vi "Calculator-V1.2.vi"() -> ()   [LabVIEW 2014]
panel:
  out "Result":dbl
  in  "Equal":bool
  in  "MUL":bool
  in  "SUB":bool
  in  "DEV":bool
  in  "SUM":bool
  in  "y":dbl
  in  "x":dbl
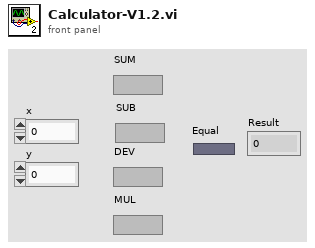
[diagram p1: front panel]
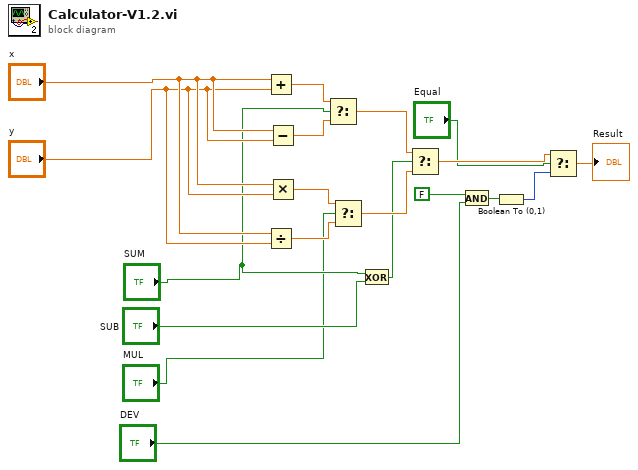
[diagram p0: block diagram]
diagram:
  n1 = Add(x="x", y="y") -> (x+y=w17:dbl)
  n2 = Divide(x="x", y="y") -> (x/y=w14:dbl)
  n3 = Subtract(x="x", y="y") -> (x-y=w16:dbl)
  n4 = Multiply(x="x", y="y") -> (x*y=w15:dbl)
  n5 = Select(t=w17, s="SUM", f=w16) -> (s? t:f=w13:dbl)
  n6 = Select(t=w15, s="MUL", f=w14) -> (s? t:f=w12:dbl)
  n7 = Exclusive Or(1:"SUB", 2:"SUM") -> (0:w9:bool)
  n8 = Select(t=w13, s=w9, f=w12) -> (s? t:f=w8:dbl)
  n9 = And(x=FALSE, y="DEV") -> (x .and. y?=w2:bool)
  n10 = Boolean To (0,1)(Boolean=w2) -> (0, 1=w1:i16)
  n11 = Select(t=w8, s="Equal", f=w1) -> (s? t:f=→"Result":dbl)
